vi "UTILITY Timeout Calc.vi"(5 "Initialize Rate":bool, 7 "Timer":dbl format="%0.2f", 10 "Gather Data Period":i32=500) -> (1 "Rate":dbl format="%0.2f", 2 "coerced(x)":i32)   [LabVIEW 2018]
uses:
  <vilib>/ptbypt/NI_PtbyPt.lvlib
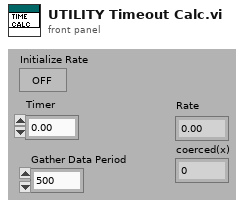
[diagram p1: front panel]
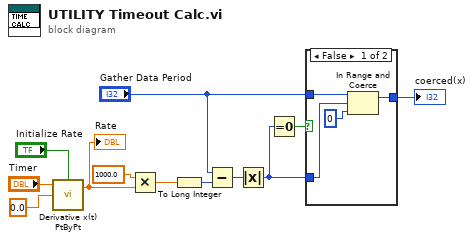
[diagram p0: block diagram]
diagram:
  n1 = call <vilib>:"Derivative x(t) PtByPt.vi"("initialize"="Initialize Rate", "initial condition"=0.0, "x"="Timer") -> ("dx/dt"=w3:dbl)  [unwired: 1 in, 1 out]
  "Rate" <- w3
  n2 = Multiply(x=1000.0, y=w3) -> (x*y=w11:dbl)
  n3 = To Long Integer(number=w11) -> (32bit integer=w9:i32)
  n4 = Subtract(x="Gather Data Period", y=w9) -> (x-y=w6:i32)
  n5 = Absolute Value(x=w6) -> (abs(x)=w5:i32)
  n6 = Equal To 0?(x=w5) -> (x = 0?=w7:bool)
  n7 = case shown="False" w7 {
    tunnel: "Gather Data Period" -> [w16 w17]
    tunnel: w5 -> [w15 _]
    tunnel: [w14 w17] -> w8
    frame False {
      n8 = In Range and Coerce(upper limit=w16, x=w15, lower limit=0) -> (coerced(x)=w14:i32)  [unwired: 1 out]
    }
    frame True {
    }
  }
  "coerced(x)" <- w8
